vi "9759 RevB Run.vi"(8 "error in":errorcluster, 10 "Period (ns)":i64, 11 "RT Data In":T1 {"Compiled Data"."9759 RevB"."Settings"."ControlCals"."ThetaLH (deg)" format="%.3f"; "Compiled Data"."9759 RevB"."Settings"."ControlCals"."ULHLag (sec)" format="%.3f"; "Compiled Data"."9759 RevB"."Settings"."ControlCals"."USLag (sec)" format="%.3f"; "Compiled Data"."9759 RevB"."Settings"."ControlCals"."TLead (sec)" format="%.3f"; "Compiled Data"."9759 RevB"."Settings"."ControlCals"."TLag (sec)" format="%.3f"}) -> (0 "error out":errorcluster, 3 "RT Data Out":T1 {"Compiled Data"."9759 RevB"."Settings"."ControlCals"."ThetaLH (deg)" format="%.3f"; "Compiled Data"."9759 RevB"."Settings"."ControlCals"."ULHLag (sec)" format="%.3f"; "Compiled Data"."9759 RevB"."Settings"."ControlCals"."USLag (sec)" format="%.3f"; "Compiled Data"."9759 RevB"."Settings"."ControlCals"."TLead (sec)" format="%.3f"; "Compiled Data"."9759 RevB"."Settings"."ControlCals"."TLag (sec)" format="%.3f"})   [LabVIEW 2015, in "NI 9759 RevB Custom Device.lvlib"]
uses:
  NI 9759 RevB Custom Device.lvlib
  Shared/Types/RT Data.ctl
  Shared/Types/Compiled Data.ctl
  Shared/Types/RT Init Data.ctl
  Shared/Types/RT Status.ctl
  Shared/Types/9759 RevB.ctl
  Shared/Types/FPGA Refs.ctl
  Shared/Types/Generic FPGA Ref.ctl
  Shared/Types/9759 RevB FPGA Ref.ctl
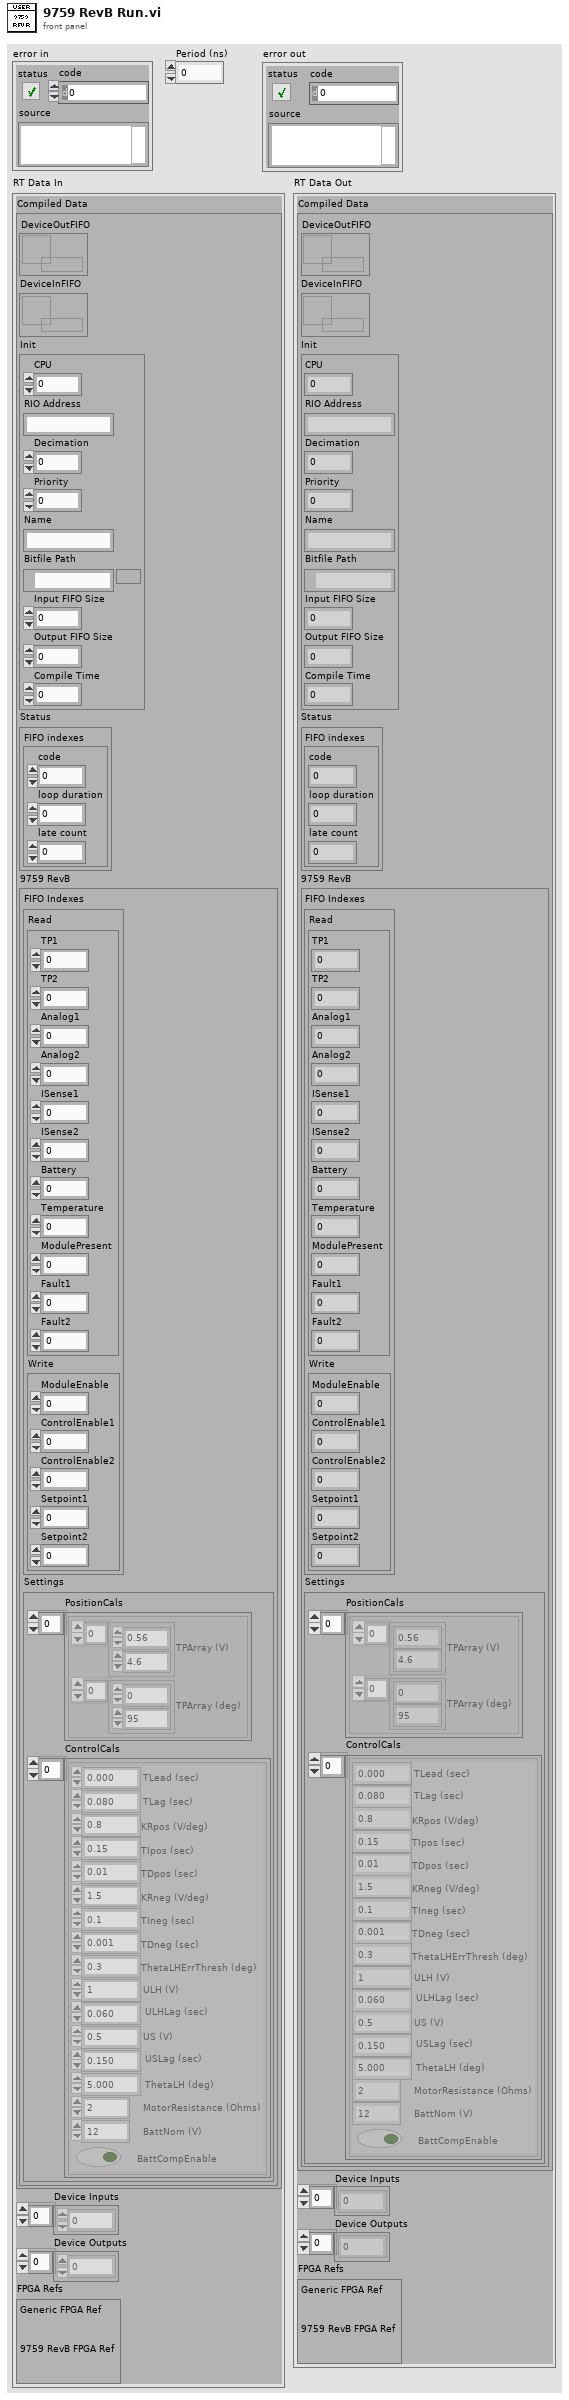
[diagram p1: front panel]
types:
  T1 = typedef "NI 9759 RevB Custom Device.lvlib/RT Data.ctl" = cluster{"Compiled Data":T2, "Device Inputs":dbl[], "Device Outputs":dbl[], "FPGA Refs":T6}
  T2 = typedef "NI 9759 RevB Custom Device.lvlib/Compiled Data.ctl" = cluster{"DeviceOutFIFO":refnum<k33>, "DeviceInFIFO":refnum<k33>, "Init":T3, "Status":T4, "9759 RevB":T5}
  T3 = typedef "NI 9759 RevB Custom Device.lvlib/RT Init Data.ctl" = cluster{"CPU":i32, "RIO Address":string, "Decimation":i32, "Priority":i32, "Name":string, "Bitfile Path":path, "Input FIFO Size":i32, "Output FIFO Size":i32, "Compile Time":dbl}
  T4 = typedef "NI 9759 RevB Custom Device.lvlib/RT Status.ctl" = cluster{"FIFO indexes":cluster{"code":i32, "loop duration":i32, "late count":i32}}
  T5 = typedef "NI 9759 RevB Custom Device.lvlib/9759 RevB.ctl" = cluster{"FIFO Indexes":cluster{"Read":cluster{"TP1":i32, "TP2":i32, "Analog1":i32, "Analog2":i32, "ISense1":i32, "ISense2":i32, "Battery":i32, "Temperature":i32, "ModulePresent":i32, "Fault1":i32, "Fault2":i32}, "Write":cluster{"ModuleEnable":i32, "ControlEnable1":i32, "ControlEnable2":i32, "Setpoint1":i32, "Setpoint2":i32}}, "Settings":cluster{"PositionCals":cluster{"TPArray (V)":sgl[], "TPArray (deg)":sgl[]}[], "ControlCals":cluster{"TLead (sec)":sgl, "TLag (sec)":sgl, "KRpos (V/deg)":sgl, "TIpos (sec)":sgl, "TDpos (sec)":sgl, "KRneg (V/deg)":sgl, "TIneg (sec)":sgl, "TDneg (sec)":sgl, "ThetaLHErrThresh (deg)":sgl, "ULH (V)":sgl, "ULHLag (sec)":sgl, "US (V)":sgl, "USLag (sec)":sgl, "ThetaLH (deg)":sgl, "MotorResistance (Ohms)":sgl, "BattNom (V)":sgl, "BattCompEnable":bool}[]}}
  T6 = typedef "NI 9759 RevB Custom Device.lvlib/FPGA Refs.ctl" = cluster{"Generic FPGA Ref":T7, "9759 RevB FPGA Ref":T8}
  T7 = typedef "NI 9759 RevB Custom Device.lvlib/Generic FPGA Ref.ctl" = refnum<k20>
  T8 = typedef "NI 9759 RevB Custom Device.lvlib/9759 RevB FPGA Ref.ctl" = refnum<k20>
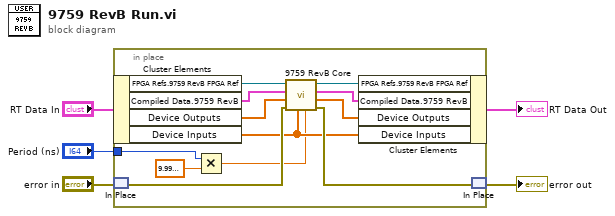
[diagram p0: block diagram]
diagram:
  n1 = in-place {
    in-place-border: "Period (ns)" -> [w8]
    n2 = in-place-cluster #1("RT Data In") -> ("FPGA Refs.9759 RevB FPGA Ref"=w17:T8, "Compiled Data.9759 RevB"=w11:T5, "Device Outputs"=w14:dbl[], "Device Inputs"=w12:dbl[])
    n3 = in-place-match #2("error in") -> (w16:errorcluster)
    n4 = Multiply(x=w8, y=sgl 1e-09) -> (x*y=w7:sgl)
    n5 = call "9759 RevB Core.vi"("dt (s)"=w7, "Device Inputs in"=w12, "error in (no error)"=w16, "Device Outputs in"=w14, "9759 RevB in"=w11, "FPGA Ref in"=w17) -> ("error out"=w15:errorcluster, "Device Outputs out"=w13:dbl[], "9759 RevB out"=w10:T5, "FPGA Ref out"=w9:T8)  [unwired: 2 in]
    n6 = in-place-cluster #1("FPGA Refs.9759 RevB FPGA Ref"=w9, "Compiled Data.9759 RevB"=w10, "Device Outputs"=w13, "Device Inputs"=w12) -> (→"RT Data Out":T1)
    n7 = in-place-match #2(w15) -> (→"error out":errorcluster)
  }
